vi "CaseStructureExamples.vi"() -> ()   [LabVIEW 2021]
panel:
  in  "a 2":bool
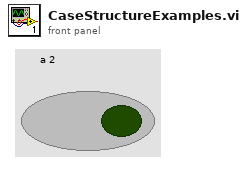
[diagram p1: front panel]
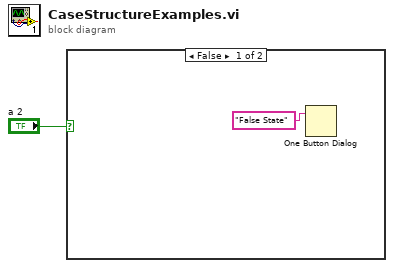
[diagram p0: block diagram]
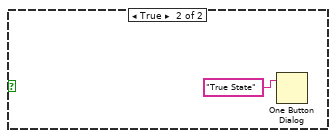
[diagram p2: hidden frame]
diagram:
  n1 = case shown="False" "a 2" {
    frame False {
      n2 = One Button Dialog(message="False State") -> ()  [unwired: 1 in, 1 out]
    }
    frame True {
      n3 = One Button Dialog(message="True State") -> ()  [unwired: 1 in, 1 out]
    }
  }
